vi "FT_Close_Device.vi"(1 "Handle":u32) -> (0 "FT_Status":u32)   [LabVIEW 2014]
uses:
  FTD2XX.DLL
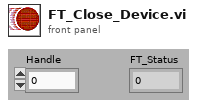
[diagram p1: front panel]
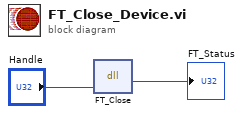
[diagram p0: block diagram]
diagram:
  n1 = dll-call lib="FTD2XX.dll" fn="FT_Close"("Handle"="Handle") -> ("FT_Status"=→"FT_Status":u32)  [unwired: 4 in, 2 out]
